vi "Run 3.vi"   [LabVIEW 2016]
types:
  T1 = typedef "LVHSConnector.ctl" = refnum<class "BrickReference.lvclass">
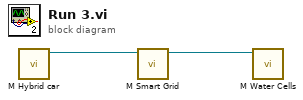
[diagram p0: block diagram]
diagram:
  n1 = call "M Hybrid car.vi"() -> ("EV3 out"=w2:T1)  [unwired: 11 in]
  n2 = call "M Smart Grid.vi"("EV3 in"=w2) -> ("EV3 out"=w1:T1)  [unwired: 10 in]
  n3 = call "M Water Cells.vi"("EV3 in"=w1) -> ()  [unwired: 11 in]
